vi "Zstack acquisition with modified signal input.vi"() -> ()   [LabVIEW 2020]
uses:
  <vilib>/DAQmx/write.llb/DAQmx Write (Analog Wfm 1Chan NSamp).vi
  <vilib>/Utility/file.llb/Read Delimited Spreadsheet (DBL).vi
  <vilib>/DAQmx/create/channels.llb/DAQmx Create Channel (AO-Voltage-Basic).vi
  <vilib>/DAQmx/configure/timing.llb/DAQmx Timing (Sample Clock).vi
  <vilib>/DAQmx/miscellaneous.llb/DAQmx Fill In Error Info.vi
  <vilib>/DAQmx/create/channels.llb/DAQmx Create Channel (CO-Pulse Generation-Frequency).vi
  <vilib>/DAQmx/configure/timing.llb/DAQmx Timing (Implicit).vi
  <resource>/objmgr/daqmx.rc
panel:
  out "Signal input":dbl[](graph)=[-0.285, -0.284, -0.284, -0.283, -0.282, -0.282, -0.281, -0.28, -0.28, -0.279, -0.278, -0.278, -0.277, -0.277, -0.276, -0.275, -0.275, -0.274, -0.273, -0.273, -0.272, -0.271, -0.271, -0.27, -0.269, -0.269, -0.268, -0.267, -0.267, -0.266, -0.266, -0.265, -0.264, -0.264, -0.263, -0.262, -0.262, -0.261, -0.26, -0.26, -0.259, -0.258, -0.258, -0.257, -0.257, -0.256, -0.255, -0.255, -0.254, -0.253, -0.253, -0.252, -0.251, -0.251, -0.25, -0.25, -0.249, -0.248, -0.248, -0.247, -0.246, -0.246, -0.245, -0.244, -0.244, -0.243, -0.243, -0.242, -0.241, -0.241, -0.24, -0.239, -0.239, -0.238, -0.237, -0.237, -0.236, -0.236, -0.235, -0.234, -0.234, -0.233, -0.232, -0.232, -0.231, -0.231, -0.23, -0.229, -0.229, -0.228, -0.227, -0.227, -0.226, -0.226, -0.225, -0.224, -0.224, -0.223, -0.222, -0.222, -0.221, -0.221, -0.22, -0.219, -0.219, -0.218, -0.218, -0.217, -0.216, -0.216, -0.215, -0.214, -0.214, -0.213, -0.213, -0.212, -0.211, -0.211, -0.21, -0.209, -0.209, -0.208, -0.208, -0.207, -0.206, -0.206, -0.205, -0.205, -0.204, -0.203, -0.203, -0.202, -0.202, -0.201, -0.2, -0.2, -0.199, -0.198, -0.198, -0.197, -0.197, -0.196, -0.195, -0.195, -0.194, -0.194, -0.193, -0.192, -0.192, -0.191, -0.191, -0.19, -0.189, -0.189, -0.188, -0.188, -0.187, -0.186, -0.186, -0.185, -0.185, -0.184, -0.183, -0.183, -0.182, -0.182, -0.181, -0.18, -0.18, -0.179, -0.179, -0.178, -0.177, -0.177, -0.176, -0.176, -0.175, -0.174, -0.174, -0.173, -0.173, -0.172, -0.171, -0.171, -0.17, -0.17, -0.169, -0.168, -0.168, -0.167, -0.167, -0.166, -0.165, -0.165, -0.164, -0.164, -0.163, -0.162, -0.162, -0.161, -0.161, -0.16, -0.16, -0.159, -0.158, -0.158, -0.157, -0.157, -0.156, -0.155, -0.155, -0.154, -0.154, -0.153, -0.153, -0.152, -0.151, -0.151, -0.15, -0.15, -0.149, -0.148, -0.148, -0.147, -0.147, -0.146, -0.146, -0.145, -0.144, -0.144, -0.143, -0.143, -0.142, -0.141, -0.141, -0.14, -0.14, -0.139, -0.139, -0.138, -0.137, -0.137, -0.136, -0.136, -0.135, -0.135, -0.134, -0.133, -0.133, -0.132, -0.132, -0.131, -0.131, -0.13, -0.129, -0.129, -0.128, -0.128, -0.127, -0.127, -0.126, -0.125, -0.125, -0.124, -0.124, -0.123, -0.123, -0.122, -0.121, -0.121, -0.12, -0.12, -0.119, -0.119, -0.118, -0.117, -0.117, -0.116, -0.116, -0.115, -0.115, -0.114, -0.114, -0.113, -0.112, -0.112, -0.111, -0.111, -0.11, -0.11, -0.109, -0.108, -0.108, -0.107, -0.107, -0.106, -0.106, -0.105, -0.105, -0.104, -0.103, -0.103, -0.102, -0.102, -0.101, -0.101, -0.1, -0.1, -0.099, -0.098, -0.098, -0.097, -0.097, -0.096, -0.096, -0.095, -0.095, -0.094, -0.094, -0.093, -0.092, -0.092, -0.091, -0.091, -0.09, -0.09, -0.089, -0.089, -0.088, -0.087, -0.087, -0.086, -0.086, -0.085, -0.085, -0.084, -0.084, -0.083, -0.083, -0.082, -0.081, -0.081, -0.08, -0.08, -0.079, -0.079, -0.078, -0.078, -0.077, -0.077, -0.076, -0.076, -0.075, -0.074, -0.074, -0.073, -0.073, -0.072, -0.072, -0.071, -0.071, -0.07, -0.07, -0.069, -0.069, -0.068, -0.067, -0.067, -0.066, -0.066, -0.065, -0.065, -0.064, -0.064, -0.063, -0.063, -0.062, -0.062, -0.061, -0.061, -0.06, -0.059, -0.059, -0.058, -0.058, -0.057, -0.057, -0.056, -0.056, -0.055, -0.055, -0.054, -0.054, -0.053, -0.053, -0.052, -0.052, -0.051, -0.051, -0.05, -0.049, -0.049, -0.048, -0.048, -0.047, -0.047, -0.046, -0.046, -0.045, -0.045, -0.044, -0.044, -0.043, -0.043, -0.042, -0.042, -0.041, -0.041, -0.04, -0.04, -0.039, -0.039, -0.038, -0.038, -0.037, -0.036, -0.036, -0.035, -0.035, -0.034, -0.034, -0.033, -0.033, -0.032, -0.032, -0.031, -0.031, -0.03, -0.03, -0.029, -0.029, -0.028, -0.028, -0.027, -0.027, -0.026, -0.026, -0.025, -0.025, -0.024, -0.024, -0.023, -0.023, -0.022, -0.022, -0.021, -0.021, -0.02, -0.02, -0.019, -0.019, -0.018, -0.018, -0.017, -0.017, -0.016, -0.016, -0.015, -0.015, -0.014, -0.014, -0.013, -0.013, -0.012, -0.012, -0.011, -0.011, -0.01, -0.01, -0.009, -0.009, -0.008, -0.008, -0.007, -0.007, -0.006, -0.006, -0.005, -0.005, -0.004, -0.004, -0.003, -0.003, -0.002, -0.002, -0.001, -0.001, 0.0, 0.0, 0.001, 0.001, 0.002, 0.002, 0.003, 0.003, 0.004, 0.004, 0.005, 0.005, 0.006, 0.006, 0.007, 0.007, 0.008, 0.008, 0.009, 0.009, 0.01, 0.01, 0.011, 0.011, 0.011, 0.012, 0.012, 0.013, 0.013, 0.014, 0.014, 0.015, 0.015, 0.016, 0.016, 0.017, 0.017, 0.018, 0.018, 0.019, 0.019, 0.02, 0.02, 0.021, 0.021, 0.022, 0.022, 0.023, 0.023, 0.023, 0.024, 0.024, 0.025, 0.025, 0.026, 0.026, 0.027, 0.027, 0.028, 0.028, 0.029, 0.029, 0.03, 0.03, 0.031, 0.031, 0.032, 0.032, 0.032, 0.033, 0.033, 0.034, 0.034, 0.035, 0.035, 0.036, 0.036, 0.037, 0.037, 0.038, 0.038, 0.039, 0.039, 0.039, 0.04, 0.04, 0.041, 0.041, 0.042, 0.042, 0.043, 0.043, 0.044, 0.044, 0.045, 0.045, 0.046, 0.046, 0.046, 0.047, 0.047, 0.048, 0.048, 0.049, 0.049, 0.05, 0.05, 0.051, 0.051, 0.051, 0.052, 0.052, 0.053, 0.053, 0.054, 0.054, 0.055, 0.055, 0.056, 0.056, 0.056, 0.057, 0.057, 0.058, 0.058, 0.059, 0.059, 0.06, 0.06, 0.061, 0.061, 0.061, 0.062, 0.062, 0.063, 0.063, 0.064, 0.064, 0.065, 0.065, 0.065, 0.066, 0.066, 0.067, 0.067, 0.068, 0.068, 0.069, 0.069, 0.069, 0.07, 0.07, 0.071, 0.071, 0.072, 0.072, 0.073, 0.073, 0.073, 0.074, 0.074, 0.075, 0.075, 0.076, 0.076, 0.077, 0.077, 0.077, 0.078, 0.078, 0.079, 0.079, 0.08, 0.08, 0.08, 0.081, 0.081, 0.082, 0.082, 0.083, 0.083, 0.083, 0.084, 0.084, 0.085, 0.085, 0.086, 0.086, 0.087, 0.087, 0.087, 0.088, 0.088, 0.089, 0.089, 0.09, 0.09, 0.09, 0.091, 0.091, 0.092, 0.092, 0.093, 0.093, 0.093, 0.094, 0.094, 0.095, 0.095, 0.095, 0.096, 0.096, 0.097, 0.097, 0.098, 0.098, 0.098, 0.099, 0.099, 0.1, 0.1, 0.101, 0.101, 0.101, 0.102, 0.102, 0.103, 0.103, 0.103, 0.104, 0.104, 0.105, 0.105, 0.106, 0.106, 0.106, 0.107, 0.107, 0.108, 0.108, 0.108, 0.109, 0.109, 0.11, 0.11, 0.111, 0.111, 0.111, 0.112, 0.112, 0.113, 0.113, 0.113, 0.114, 0.114, 0.115, 0.115, 0.115, 0.116, 0.116, 0.117, 0.117, 0.117, 0.118, 0.118, 0.119, 0.119, 0.12, 0.12, 0.12, 0.121, 0.121, 0.122, 0.122, 0.122, 0.123, 0.123, 0.124, 0.124, 0.124, 0.125, 0.125, 0.126, 0.126, 0.126, 0.127, 0.127, 0.128, 0.128, 0.128, 0.129, 0.129, 0.13, 0.13, 0.13, 0.131, 0.131, 0.132, 0.132, 0.132, 0.133, 0.133, 0.133, 0.134, 0.134, 0.135, 0.135, 0.135, 0.136, 0.136, 0.137, 0.137, 0.137, 0.138, 0.138, 0.139, 0.139, 0.139, 0.14, 0.14, 0.141, 0.141, 0.141, 0.142, 0.142, 0.142, 0.143, 0.143, 0.144, 0.144, 0.144, 0.145, 0.145, 0.146, 0.146, 0.146, 0.147, 0.147, 0.147, 0.148, 0.148, 0.149, 0.149, 0.149, 0.15, 0.15, 0.15, 0.151, 0.151, 0.152, 0.152, 0.152, 0.153, 0.153, 0.154, 0.154, 0.154, 0.155, 0.155, 0.155, 0.156, 0.156, 0.157, 0.157, 0.157, 0.158, 0.158, 0.158, 0.159, 0.159, 0.159, 0.16, 0.16, 0.161, 0.161, 0.161, 0.162, 0.162, 0.162, 0.163, 0.163, 0.164, 0.164, 0.164, 0.165, 0.165, 0.165, 0.166, 0.166, 0.166, 0.167, 0.167, 0.168, 0.168, 0.168, 0.169, 0.169, 0.169, 0.17, 0.17, 0.17, 0.171, 0.171, 0.172, 0.172, 0.172, 0.173, 0.173, 0.173, 0.174, 0.174, 0.174, 0.175, 0.175, 0.176, 0.176, 0.176, 0.177, 0.177, 0.177, 0.178, 0.178, 0.178, 0.179, 0.179, 0.179, 0.18, 0.18, 0.18, 0.181, 0.181, 0.182, 0.182, 0.182, 0.183, 0.183, 0.183, 0.184, 0.184, 0.184, 0.185, 0.185, 0.185, 0.186, 0.186, 0.186, 0.187, 0.187, 0.187, 0.188, 0.188, 0.189, 0.189, 0.189, 0.19, 0.19, 0.19, 0.191, 0.191, 0.191, 0.192, 0.192, 0.192, 0.193, 0.193, 0.193, 0.194, 0.194, 0.194, 0.195, 0.195, 0.195, 0.196, 0.196, 0.196, 0.197, 0.197, 0.197, 0.198, 0.198, 0.198, 0.199, 0.199, 0.199, 0.2, 0.2, 0.2, 0.201, 0.201, 0.201, 0.202, 0.202, 0.202, 0.203, 0.203, 0.203, 0.204, 0.204, 0.204, 0.205, 0.205, 0.205, 0.206]
  out "actual frequency":dbl=10.0
  in  "stop":bool
  out "# Samples written per channel":u32=1000
  out "Error out":errorcluster
  in  "Disable Axis":bool
  in  "Z step size (um)":dbl=0.2
  out "Number of Slices":dbl=100.0
  in  "Input will be multiplied by 5":dbl=20.0
  in  "file path (dialog if empty) 2":path=path "C:/Users/htm22/Downloads/Voice coil input.txt"
  in  "Acquire Z Stack?":bool=TRUE
  out "GetFirmwareVersion 2":string="3.03\r"
  out "Connected":bool=TRUE
  in  "SPIIPLUSCOM660Lib.IAsyncChannel":refnum<k7>
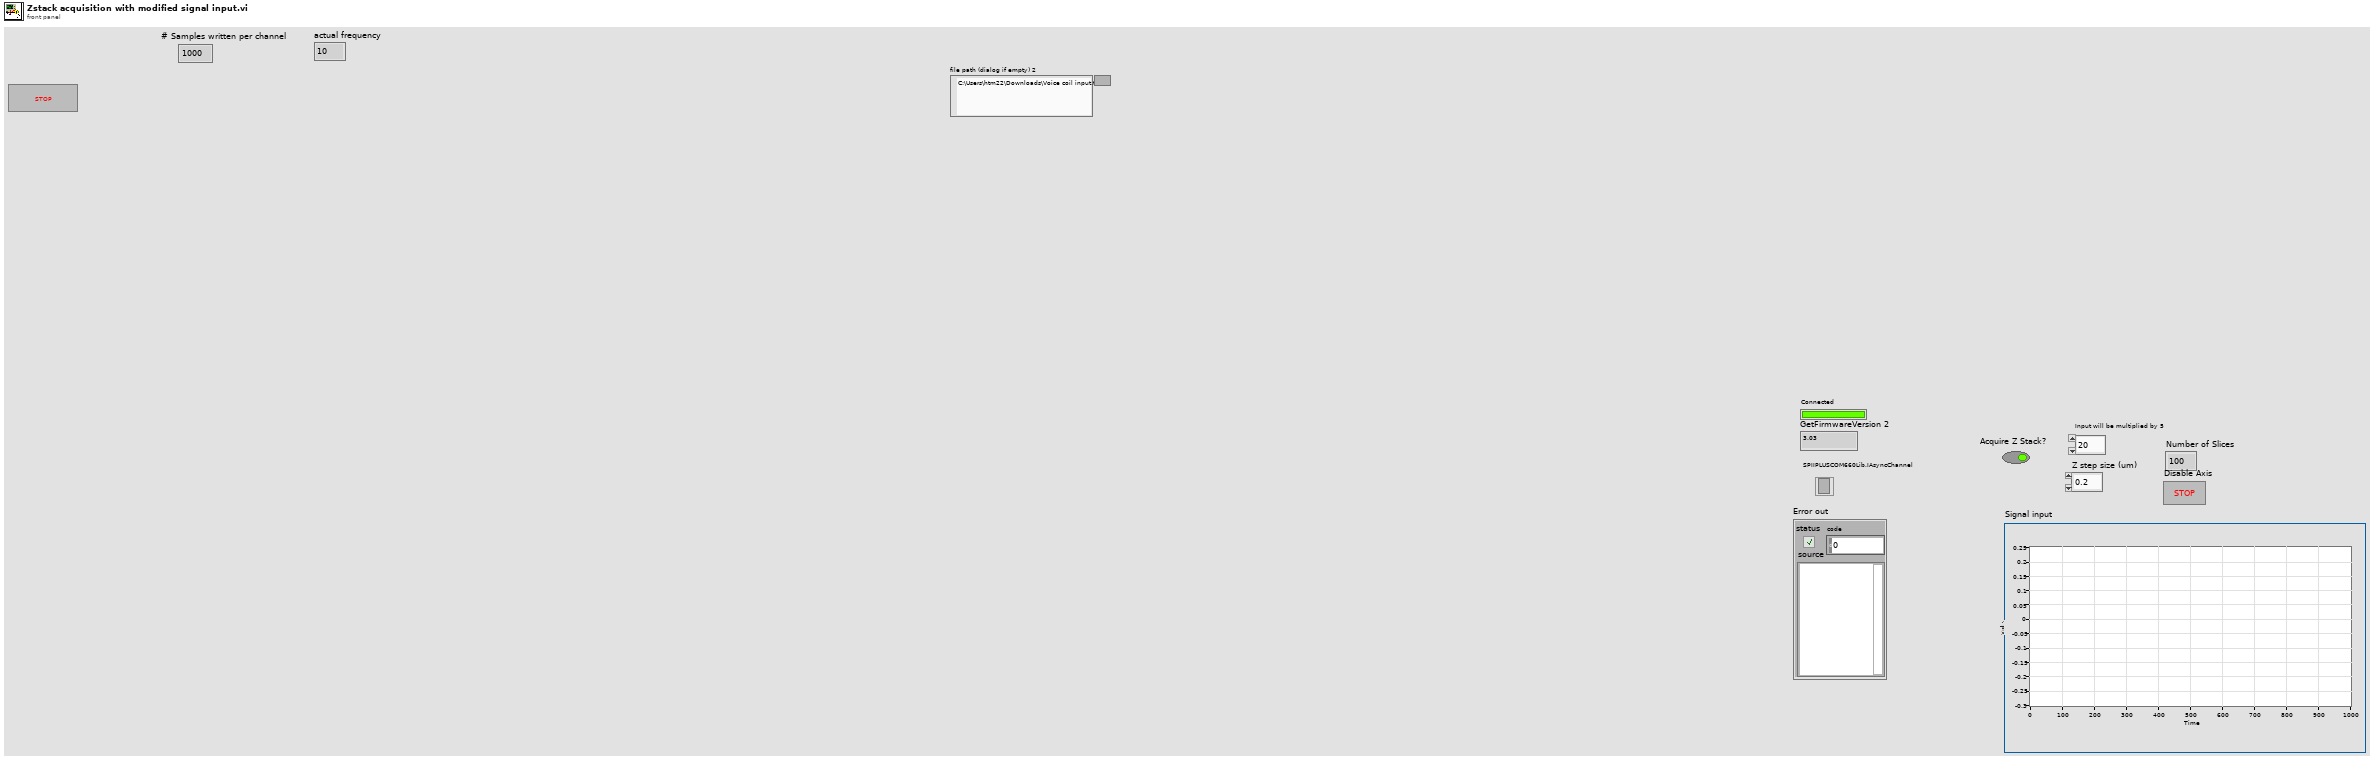
[diagram p1: front panel]
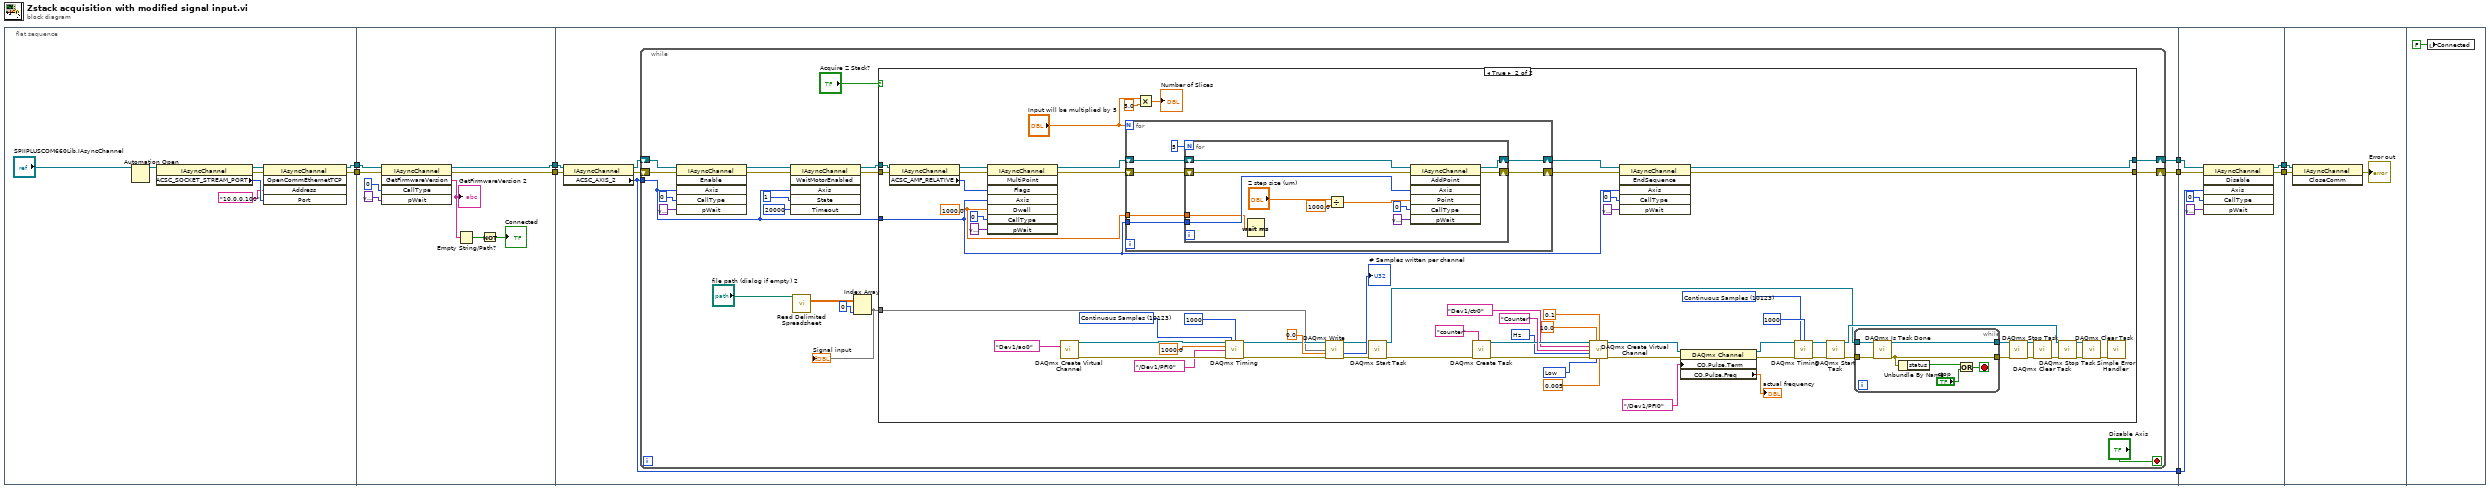
[diagram p0: block diagram]
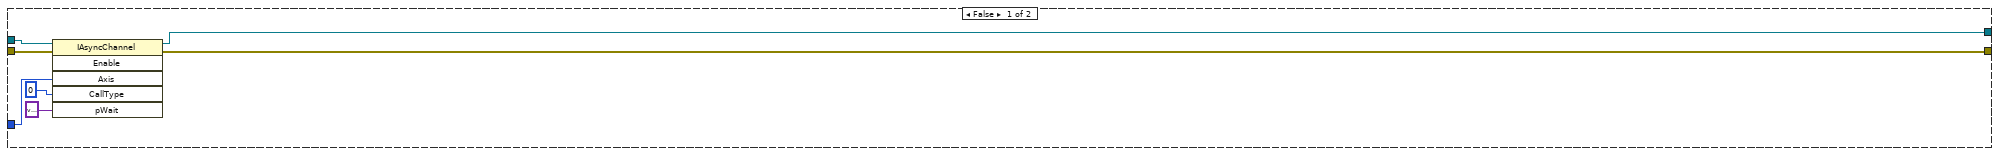
[diagram p2: hidden frame]
diagram:
  n1 = flat-sequence {
    tunnel: [w12] -> w9
    tunnel: [w11] -> w8
    tunnel: w9 -> [w22]
    tunnel: w8 -> [w21]
    tunnel: [w19] -> w7
    tunnel: [w18] -> w6
    tunnel: w7 -> [w31]
    tunnel: w6 -> [w30]
    tunnel: [w33] -> w5
    tunnel: [w32] -> w4
    tunnel: [w29] -> w3
    tunnel: w5 -> [w157]
    tunnel: w4 -> [w156]
    tunnel: [w155] -> w2
    tunnel: [w154] -> w1
    tunnel: w3 -> [w153]
    tunnel: w2 -> [w159]
    tunnel: w1 -> [w158]
    frame #0 {
      n2 = Automation Open(Automation Refnum="SPIIPLUSCOM660Lib.IAsyncChannel") -> (Automation Refnum=w17:refnum<k7>)  [unwired: 3 in, 1 out]
      n3 = property class="IAsyncChannel"(reference=w17) -> (reference out=w16:refnum<k7>, error out=w10:errorcluster, "ACSC_SOCKET_STREAM_PORT"=w14:i32)  [unwired: 1 in]
      n4 = invoke class="IAsyncChannel" method="OpenCommEthernetTCP"(reference=w16, error in=w10, "Address"="10.0.0.100", "Port"=w14) -> (reference out=w12:refnum<k7>, error out=w11:errorcluster)  [unwired: 1 in, 3 out]
    }
    frame #1 {
      n5 = invoke class="IAsyncChannel" method="GetFirmwareVersion"(reference=w22, error in=w21, "CallType"=u64 0, "pWait"=variant) -> (reference out=w19:refnum<k7>, error out=w18:errorcluster, "GetFirmwareVersion"=w24:string)  [unwired: 1 in, 2 out]
      "GetFirmwareVersion 2" <- w24
      n6 = Empty String/Path?(string/path=w24) -> (empty?=w23:bool)
      n7 = Not(x=w23) -> (.not. x?=→"Connected":bool)
    }
    frame #2 {
      n8 = property class="IAsyncChannel"(reference=w31, error in=w30) -> (reference out=w28:refnum<k7>, error out=w27:errorcluster, "ACSC_AXIS_2"=w29:i32)
      n9 = while {
        shift-right: [w52] -> w33
        shift-left: w28 -> [w44]
        shift-right: [w51] -> w32
        shift-left: w27 -> [w43]
        tunnel: w29 -> [w40]
        stop <- "Disable Axis" stop-if-true
        n10 = invoke class="IAsyncChannel" method="Enable"(reference=w44, error in=w43, "Axis"=w40, "CallType"=u64 0, "pWait"=variant) -> (reference out=w48:refnum<k7>, error out=w47:errorcluster)  [unwired: 1 in, 4 out]
        n11 = invoke class="IAsyncChannel" method="WaitMotorEnabled"(reference=w48, error in=w47, "Axis"=w40, "State"=1, "Timeout"=20000) -> (reference out=w39:refnum<k7>, error out=w38:errorcluster)  [unwired: 1 in, 4 out]
        n12 = call-poly <vilib>:"Read Delimited Spreadsheet.vi"("file path (dialog if empty)"="file path (dialog if empty) 2") -> ("all rows"=w35:dbl[][])  [unwired: 9 in, 5 out]
        n13 = Index Array(array=w35, index (col)=0 ("dimension size")) -> (element=w34:dbl[])  [unwired: 1 in]
        "Signal input" <- w34
        n14 = case shown="True" "Acquire Z Stack?" {
          tunnel: w39 -> [w59 w113]
          tunnel: w38 -> [w58 w114]
          tunnel: [w57 w111] -> w52
          tunnel: [w56 w112] -> w51
          tunnel: w40 -> [w55 w110]
          tunnel: w34 -> [_ w68]
          frame False {
            n15 = invoke class="IAsyncChannel" method="Enable"(reference=w59, error in=w58, "Axis"=w55, "CallType"=u64 0, "pWait"=variant) -> (reference out=w57:refnum<k7>, error out=w56:errorcluster)  [unwired: 1 in, 4 out]
          }
          frame True {
            w63 = 10123 items=["Finite Samples"=10178, "Continuous Samples"=10123, "Hardware Timed Single Point"=12522] ("sample mode")
            w72 = 10214 items=["High"=10192, "Low"=10214] ("idle state")
            w73 = 10373 items=["Hz"=10373] ("units")
            w103 = 10123 items=["Finite Samples"=10178, "Continuous Samples"=10123, "Hardware Timed Single Point"=12522] ("sample mode")
            w106 = 1000.0 ("Exposure time (ms)")
            n16 = property class="IAsyncChannel"(reference=w113, error in=w114) -> (reference out=w123:refnum<k7>, error out=w122:errorcluster, "ACSC_AMF_RELATIVE"=w119:i32)
            n17 = invoke class="IAsyncChannel" method="MultiPoint"(reference=w123, error in=w122, "Flags"=w119, "Axis"=w110, "Dwell"=w106, "CallType"=u64 0, "pWait"=variant) -> (reference out=w118:refnum<k7>, error out=w117:errorcluster)  [unwired: 1 in, 6 out]
            n18 = call-poly <vilib>:"DAQmx Create Virtual Channel.vi"("physical channels"=tag "Dev1/ao0") -> ("task out"=w105:refnum<k21>, "error out"=w104:errorcluster)  [unwired: 13 in]
            n19 = for {
              N: "Input will be multiplied by 5" -> [_]
              tunnel: w110 -> [w135]
              tunnel: w106 -> [w134]
              shift-right: [w137] -> w116
              shift-left: w118 -> [w139]
              shift-right: [w136] -> w115
              shift-left: w117 -> [w138]
              n20 = for {
                N: 5 -> [_]
                tunnel: w135 -> [w150]
                shift-right: [w145] -> w137
                shift-left: w139 -> [w149]
                shift-right: [w144] -> w136
                shift-left: w138 -> [w148]
                tunnel: w134 -> [w140]
                n21 = Wait (ms)(milliseconds to wait=w140) -> ()  [unwired: 1 out]
                n22 = Divide(x="Z step size (um)", y=1000.0) -> (x/y=w141:dbl)
                n23 = invoke class="IAsyncChannel" method="AddPoint"(reference=w149, error in=w148, "Axis"=w150, "Point"=w141, "CallType"=u64 0, "pWait"=variant) -> (reference out=w145:refnum<k7>, error out=w144:errorcluster)  [unwired: 1 in, 5 out]
              }
            }
            n24 = Multiply(x="Input will be multiplied by 5", y=5.0) -> (x*y=→"Number of Slices":dbl)
            n25 = call-poly <vilib>:"DAQmx Timing.vi"("task/channels in"=w105, "sample mode"=w103, "samples per channel"=1000, "rate"=1000.0, "source"=tag "/Dev1/PFI0", "error in"=w104) -> ("task out"=w70:refnum<k21>, "error out"=w69:errorcluster)  [unwired: 8 in]
            n26 = call-poly <vilib>:"DAQmx Write.vi"("task/channels in"=w70, "data"=w68, "timeout"=0.0, "error in"=w69) -> ("task out"=w66:refnum<k21>, "number of samples written per channel"=→"# Samples written per channel":u32, "error out"=w65:errorcluster)  [unwired: 9 in]
            n27 = call <vilib>:"DAQmx Start Task.vi"("task/channels in"=w66, "error in"=w65) -> ("task out"=w62:refnum<k21>, "error out"=w64:errorcluster)  [unwired: 12 in]
            n28 = call <vilib>:"DAQmx Create Task.vi"("new task name"="counter", "error in"=w64) -> ("task out"=w97:refnum<k21>, "error out"=w95:errorcluster)  [unwired: 12 in]
            n29 = call-poly <vilib>:"DAQmx Create Virtual Channel.vi"("task in"=w97, "frequency"=10.0, "duty cycle"=0.1, "counter"=tag "Dev1/ctr0", "name to assign"="Counter", "units"=w73, "error in"=w95, "idle state"=w72, "initial delay"=0.005) -> ("task out"=w94:refnum<k21>, "error out"=w93:errorcluster)  [unwired: 5 in]
            n30 = invoke class="IAsyncChannel" method="EndSequence"(reference=w116, error in=w115, "Axis"=w110, "CallType"=u64 0, "pWait"=variant) -> (reference out=w111:refnum<k7>, error out=w112:errorcluster)  [unwired: 1 in, 4 out]
            n31 = property class="DAQmx Channel"(reference=w94, error in=w93, "CO.Pulse.Term"=tag "/Dev1/PFI0") -> (reference out=w90:refnum<k21>, error out=w91:errorcluster, "CO.Pulse.Freq"=→"actual frequency":dbl)
            n32 = call-poly <vilib>:"DAQmx Timing.vi"("task/channels in"=w90, "sample mode"=w63, "samples per channel"=1000, "error in"=w91) -> ("task out"=w100:refnum<k21>, "error out"=w99:errorcluster)  [unwired: 10 in]
            n33 = call <vilib>:"DAQmx Start Task.vi"("task/channels in"=w100, "error in"=w99) -> ("task out"=w89:refnum<k21>, "error out"=w80:errorcluster)  [unwired: 12 in]
            n34 = while {
              tunnel: w62 -> [w132]
              tunnel: w80 -> [w131]
              tunnel: [w130] -> w85
              tunnel: [w129] -> w86
              stop <- w126 stop-if-true
              n35 = call <vilib>:"DAQmx Is Task Done.vi"("task/channels in"=w132, "error in"=w131) -> ("task out"=w130:refnum<k21>, "error out"=w129:errorcluster)  [unwired: 11 in, 1 out]
              n36 = Unbundle By Name(w129) -> ("status"=w128:bool)
              n37 = Or(x=w128, y="stop") -> (x .or. y?=w126:bool)
            }
            n38 = call <vilib>:"DAQmx Stop Task.vi"("task/channels in"=w85, "error in"=w86) -> ("task out"=w84:refnum<k21>, "error out"=w83:errorcluster)  [unwired: 12 in]
            n39 = call <vilib>:"DAQmx Clear Task.vi"("task in"=w84, "error in"=w83) -> ("error out"=w82:errorcluster)  [unwired: 13 in]
            n40 = call <vilib>:"DAQmx Stop Task.vi"("task/channels in"=w89, "error in"=w82) -> ("task out"=w87:refnum<k21>, "error out"=w88:errorcluster)  [unwired: 12 in]
            n41 = call <vilib>:"DAQmx Clear Task.vi"("task in"=w87, "error in"=w88) -> ("error out"=w81:errorcluster)  [unwired: 13 in]
            n42 = call <vilib>:"Simple Error Handler.vi"("error in (no error)"=w81) -> ()  [unwired: 4 in, 5 out]
          }
        }
      }
    }
    frame #3 {
      n43 = invoke class="IAsyncChannel" method="Disable"(reference=w157, error in=w156, "Axis"=w153, "CallType"=u64 0, "pWait"=variant) -> (reference out=w155:refnum<k7>, error out=w154:errorcluster)  [unwired: 1 in, 4 out]
    }
    frame #4 {
      n44 = invoke class="IAsyncChannel" method="CloseComm"(reference=w159, error in=w158) -> (error out=→"Error out":errorcluster)  [unwired: 1 in, 2 out]
    }
    frame #5 {
      n45 = local write "Connected"(FALSE ("Connected")) -> ()
    }
  }
